vi "Magazine_Execute.vi"() -> ()   [LabVIEW 2019]
uses:
  Magazine_Cluster.ctl
  Magazine_States.ctl
  <vilib>/Rock Robotics/WPI/ThirdParty/REV Robotics/SPARK MAX/Typedef/Spark MAX Control Type.ctl
  Globals/Magazine_Globals.vi
  Globals/Sensor_Values.vi
  Globals/Flywheel_Globals.vi
panel:
  out "Waveform Chart":T1(graph)
  in  "Firing_Speed":dbl=0.6
  in  "Max Magazine Speed":dbl=3300.0
  in  "Unjam_Speed":dbl=-0.2
  in  "Loading_Speed":dbl=1.0
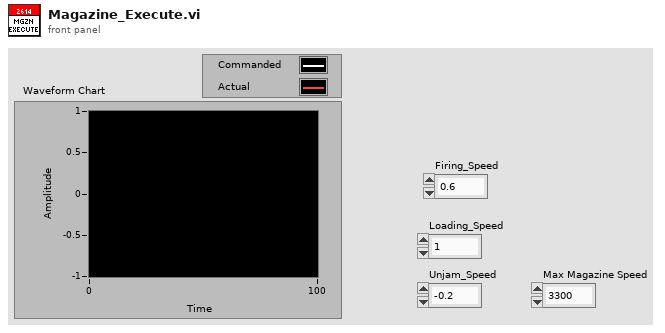
[diagram p1: front panel]
types:
  T1 = cluster{"Firing_Speed":dbl, "Magazine_Velocity(RPM)":dbl}
  T2 = typedef "WPI_MotorControlDeviceRef.ctl" = cluster{"DeviceStatus":errorcluster, "Type":T3, "PWM":cluster{"PWM Channel":T4, "DeadBand":T5}, "CAN":cluster{"Device Number":u8, "SetOutput VI Ref":variant, "GetOutput VI Ref":variant, "Enable VI Ref":variant, "Disable VI Ref":variant, "Data":variant}, "Invert":bool, "DIO PWM":cluster{"PWM \"Enable\" Channel":T4, "DIOChannel":T6, "PWM Rate":dbl}}
  T3 = typedef "WPI_MotorControlType.ctl" = enum16{"PWM", "CAN", "DIO PWM"}
  T4 = typedef "FPGA_DIOPWMChannel.ctl" = enum8{"PWM 0", "PWM 1", "PWM 2", "PWM 3", "PWM 4", "PWM 5", "PWM 6", "PWM 7", "PWM 8", "PWM 9", "PWM MXP 0", "PWM MXP 1", "PWM MXP 2", "PWM MXP 3", "PWM MXP 4", "PWM MXP 5", "PWM MXP 6", "PWM MXP 7", "PWM MXP 8", "PWM MXP 9", "Invalid"}
  T5 = typedef "WPI_PWMDeadband.ctl" = cluster{"Name":string, "maxPositivePwm":i32, "minPositivePwm":i32, "centerPwm":i32, "maxNegativePwm":i32, "minNegativePwm":i32, "angularRange":u16}
  T6 = typedef "FPGA_DIOChannel.ctl" = enum8{"DIO 0", "DIO 1", "DIO 2", "DIO 3", "DIO 4", "DIO 5", "DIO 6", "DIO 7", "DIO 8", "DIO 9", "DIO MXP 0", "DIO MXP 1", "DIO MXP 2", "DIO MXP 3", "DIO MXP 4", "DIO MXP 5", "DIO MXP 6", "DIO MXP 7", "DIO MXP 8", "DIO MXP 9", "DIO MXP 10", "DIO MXP 11", "DIO MXP 12", "DIO MXP 13", "DIO MXP 14", "DIO MXP 15", "SPI Port CS1", "SPI Port CS2", "SPI Port CS3", "SPI Port MISO", "SPI Port MOSI", "Invalid"}
  T7 = typedef "Magazine_Cluster.ctl" = cluster{"Fire":bool, "Magazine_Throttle":dbl, "Control_States":T8, "Auto_Notifier":refnum<notifier>, "Parameter_1":dbl, "Parameter_2":dbl, "Step":dbl}
  T8 = typedef "Magazine_States.ctl" = enum16{"No-Op", "Loading", "Fire", "Unjam", "Manual_Percent_Voltage", "Manual_Speed_Control", "Command_Fire"}
  T9 = typedef "Spark MAX Control Type.ctl" = enum16{"Percent VBus", "Voltage", "Velocity", "Position", "Smart Motion", "Current", "Smart Velocity"}
  T10 = cluster{"Magazine_Throttle":dbl, "Magazine_Velocity(RPM)":dbl}
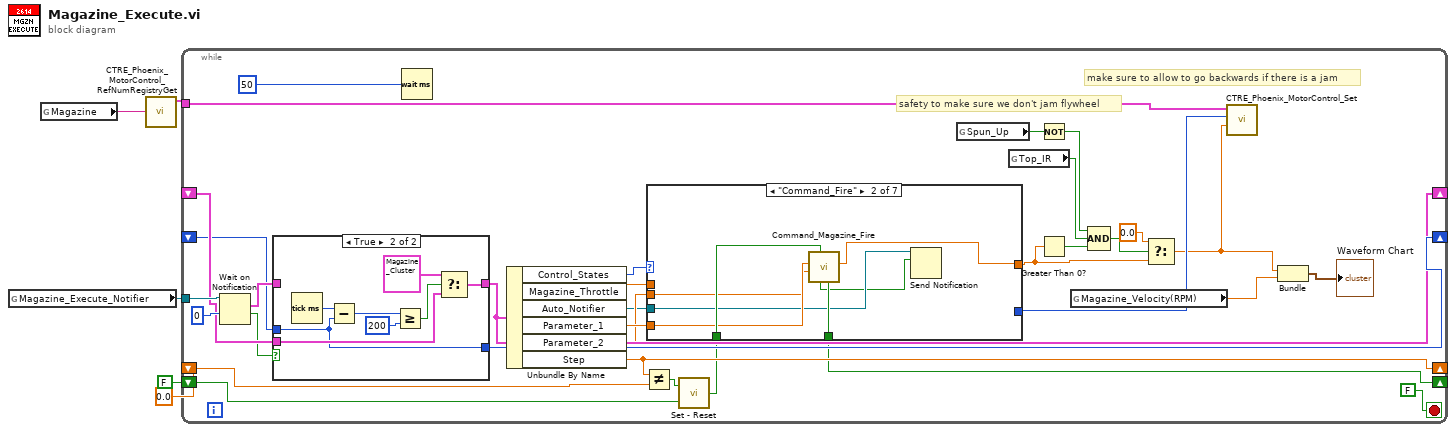
[diagram p0: block diagram]
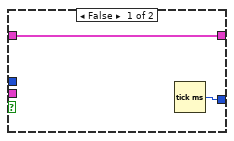
[diagram p2: hidden frame]
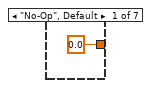
[diagram p3: hidden frame]
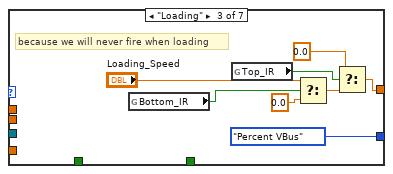
[diagram p4: hidden frame]
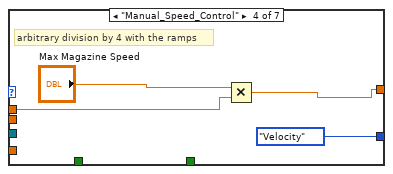
[diagram p5: hidden frame]
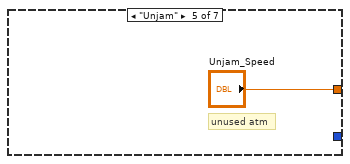
[diagram p6: hidden frame]
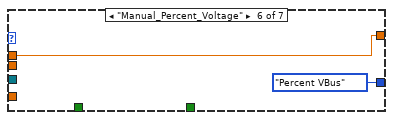
[diagram p7: hidden frame]
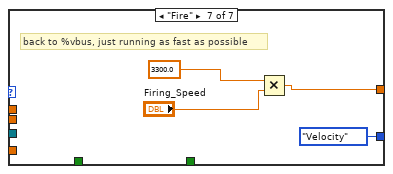
[diagram p8: hidden frame]
diagram:
  n1 = global read "Magazine_Globals.vi" "Magazine_Execute_Notifier"() -> (w5:refnum<notifier>)
  n2 = global read "Magazine_Globals.vi" "Magazine"() -> (w4:string)
  n3 = call <vilib>:"CTRE_Phoenix_MotorControl_RefNumRegistryGet.vi"("refnum name"=w4) -> ("PhoenixMotorControlDevRef"=w3:T2)  [unwired: 9 in, 1 out]
  n4 = while {
    tunnel: w5 -> [w37]
    tunnel: w3 -> [w26]
    shift-right: [w22] -> _
    shift-left: _ -> [w19]
    shift-right: [w21] -> _
    shift-left: _ -> [w20]
    shift-right: [w14] -> _
    shift-left: 0.0 ("Step") -> [w13]
    shift-right: [w10] -> _
    shift-left: FALSE ("Reint") -> [w9]
    stop <- FALSE stop-if-true
    # "make sure to allow to go backwards if there is a jam"
    # "safety to make sure we don't jam flywheel"
    n5 = Wait on Notification(notifier=w37, timeout in ms (-1)=0) -> (notification=w24:T7, timed out?=w18:bool)  [unwired: 2 in, 2 out]
    n6 = case shown="True" w18 {
      tunnel: w24 -> [w40 _]
      tunnel: [w40 w48] -> w21
      tunnel: [w39 w41] -> w22
      tunnel: w20 -> [_ w47]
      tunnel: w19 -> [_ w41]
      frame False {
        n7 = Tick Count (ms)() -> (millisecond timer value=w39:u32)
      }
      frame True {
        n8 = Tick Count (ms)() -> (millisecond timer value=w46:u32)
        n9 = Subtract(x=w46, y=w41) -> (x-y=w45:u32)
        n10 = Greater Or Equal?(x=w45, y=u32 200) -> (x >= y?=w43:bool)
        n11 = Select(t=T7 {"Fire"=FALSE, "Magazine_Throttle"=0.0, "Control_States"=enum."No-Op", "Auto_Notifier"=refnum, "Parameter_1"=0.0, "Parameter_2"=0.0, "Step"=0.0}, s=w43, f=w47) -> (s? t:f=w48:T7)
      }
    }
    n12 = Wait (ms)(milliseconds to wait=u32 50) -> ()  [unwired: 1 out]
    n13 = Unbundle By Name(w21) -> ("Control_States"=w36:T8, "Magazine_Throttle"=w35:dbl, "Auto_Notifier"=w6:refnum<notifier>, "Parameter_1"=w8:dbl, "Parameter_2"=w7:dbl, "Step"=w14:dbl)
    n14 = Not Equal?(x=w14, y=w13) -> (x != y?=w12:bool)
    n15 = call "Set - Reset.vi"("Reset"=w9, "Set"=w12) -> ("Output"=w11:bool)
    n16 = case shown="\"Command_Fire\"" w36 {
      tunnel: w35 -> [_ _ _ w66 _ w71 _]
      tunnel: [0.0 ("Magazine_Throttle") w50 w59 w65 "Unjam_Speed" w71 w72] -> w31
      tunnel: [_ _ Spark_MAX_Control_Type."Percent VBus" ("Control Mode") Spark_MAX_Control_Type."Velocity" ("Control Mode") _ Spark_MAX_Control_Type."Percent VBus" ("Control Mode") Spark_MAX_Control_Type."Velocity" ("Control Mode")] -> w25
      tunnel: w11 -> [_ w56 _ _ _ _ _]
      tunnel: [_ w55 _ _ _ _ _] -> w10
      tunnel: w8 -> [_ w54 _ _ _ _ _]
      tunnel: w7 -> [_ w53 _ _ _ _ _]
      tunnel: w6 -> [_ w52 _ _ _ _ _]
      frame "No-Op", Default {
      }
      frame "Command_Fire" {
        n17 = call "Command_Magazine_Fire.vi"("Startup"=w56, "Timeout"=w53, "Speed"=w54) -> ("Magazine_Output"=w50:dbl, "Reint"=w55:bool, "Completed"=w51:bool)  [unwired: 6 in]
        n18 = Send Notification(notification=w51, notifier=w52) -> ()  [unwired: 1 in, 2 out]
      }
      frame "Loading" {
        # "because we will never fire when loading"
        n19 = global read "Sensor_Values.vi" "Bottom_IR"() -> (w63:bool)
        n20 = global read "Sensor_Values.vi" "Top_IR"() -> (w58:bool)
        n21 = Select(t="Loading_Speed", s=w63, f=0.0 ("t")) -> (s? t:f=w60:dbl)
        n22 = Select(t=0.0, s=w58, f=w60) -> (s? t:f=w59:dbl)
      }
      frame "Manual_Speed_Control" {
        # "arbitrary division by 4 with the ramps"
        n23 = Multiply(x="Max Magazine Speed", y=w66) -> (x*y=w65:dbl)
      }
      frame "Unjam" {
        # "unused atm"
      }
      frame "Manual_Percent_Voltage" {
      }
      frame "Fire" {
        # "back to %vbus, just running as fast as possible"
        n24 = Multiply(x=3300.0, y="Firing_Speed") -> (x*y=w72:dbl)
      }
    }
    n25 = global read "Flywheel_Globals.vi" "Spun_Up"() -> (w27:bool)
    n26 = global read "Sensor_Values.vi" "Top_IR"() -> (w28:bool)
    n27 = Not(x=w27) -> (.not. x?=w33:bool)
    n28 = Greater Than 0?(x=w31) -> (x > 0?=w30:bool)
    n29 = global read "Sensor_Values.vi" "Magazine_Velocity(RPM)"() -> (w15:dbl)
    n30 = Compound Arithmetic op=AND(w33, w28, w30) -> (w32:bool)
    n31 = Select(t=0.0, s=w32, f=w31) -> (s? t:f=w17:dbl)
    n32 = call <vilib>:"CTRE_Phoenix_MotorControl_Set.vi"("Output"=w17, "Control Mode"=w25, "PhoenixMotorControlDevRef"=w26) -> ()  [unwired: 7 in, 2 out]
    n33 = Bundle("Magazine_Throttle"=w17, "Magazine_Velocity(RPM)"=w15) -> (→"Waveform Chart":T10)  [unwired: 1 in]
  }
